vi "TwGetStickSpectrumFromShMem.vi"(4 "BufIndex":i32, 5 "error in (no error)":errorcluster, 6 "SegmentEndIndex":i32, 7 "SegmentIndex":i32, 8 "Masses in":sgl[](array[numeric]), 9 "Stick spectrum in":sgl[](array[numeric])) -> (0 "Masses out":sgl[](array[numeric]), 1 "Stick spectrum out":sgl[](array[numeric]), 3 "error out":errorcluster)   [LabVIEW 2009]
uses:
  TofDaqDll.dll
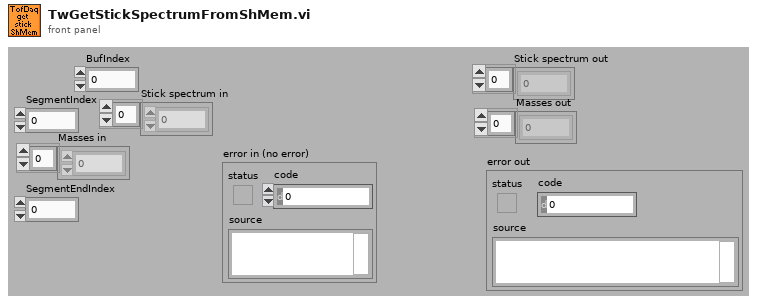
[diagram p1: front panel]
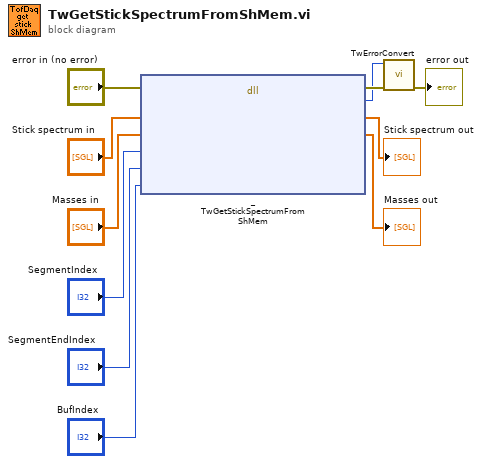
[diagram p0: block diagram]
diagram:
  n1 = dll-call lib="C:/src/TofDaq/APIandWrappers/LabView/TofDaqDll/TofDaqDll.dll" fn="_TwGetStickSpectrumFromShMem"(error in="error in (no error)", "Spectrum"="Stick spectrum in", "Masses"="Masses in", "SegmentIndex"="SegmentIndex", "SegmentEndIndex"="SegmentEndIndex", "BufIndex"="BufIndex") -> (error out=w10:errorcluster, "TwRetVal"=w9:i32, "Spectrum"=→"Stick spectrum out":sgl[], "Masses"=→"Masses out":sgl[])  [unwired: 5 in, 1 out]
  n2 = call "TwErrorConvert.vi"("error in (no error)"=w10, "error code"=w9) -> ("error out"=→"error out":errorcluster)  [unwired: 9 out]
